vi "Read PDU Resp.vi"(8 "error in (no error)":errorcluster, 11 "MB_ADU in":refnum<class "MB_ADU.lvclass">) -> (0 "error out":errorcluster, 2 "PDU":T1, 3 "MB_ADU out":refnum<class "MB_ADU.lvclass">)   [LabVIEW 2012, in "MB Master.lvlib" / "MB_ADU.lvclass"]
uses:
  MB_ADU.lvclass
  MB_PDU/MB_PDU_Cluster.ctl
  MB_ADU.lvclass/MB_ADU.ctl
  MB Master.lvlib
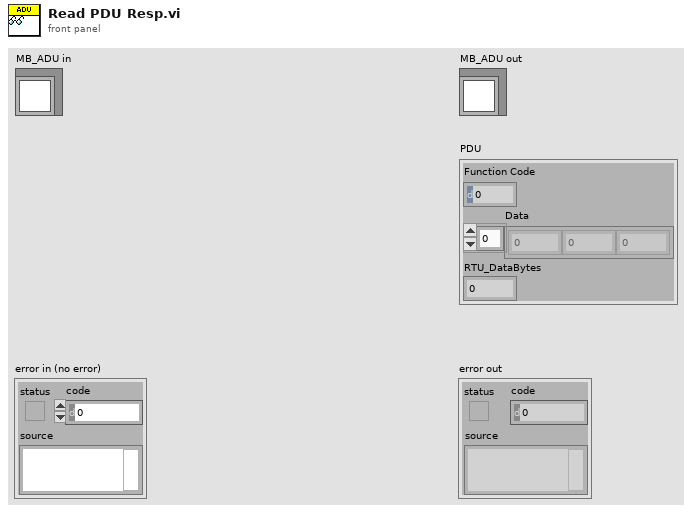
[diagram p1: front panel]
types:
  T1 = typedef "MB Master.lvlib/MB_PDU_Cluster.ctl" = cluster{"Function Code":u8, "Data":u8[], "RTU_DataBytes":i32}
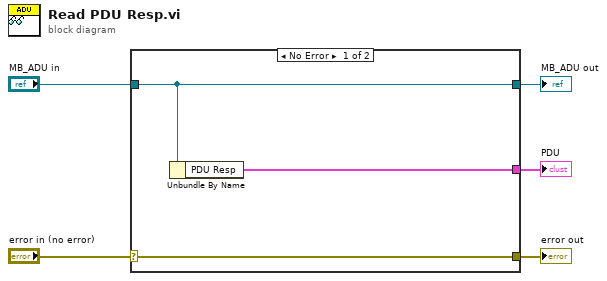
[diagram p0: block diagram]
diagram:
  n1 = case shown="No Error" "error in (no error)" {
    selector: "error in (no error)" -> [w8 w9]
    tunnel: [w8 w9] -> w4
    tunnel: [w7 w10] -> w2
    tunnel: "MB_ADU in" -> [w7 w10]
    tunnel: [w6 _] -> w1
    frame No Error {
      n2 = Unbundle By Name(w7) -> ("PDU Resp"=w6:T1)
    }
    frame Error {
    }
  }
  "error out" <- w4
  "MB_ADU out" <- w2
  "PDU" <- w1
